vi "SCLN_GetResponseFromOldServer.vi"(2 "error in (no error)":errorcluster, 3 "Index for Server":i32) -> (0 "error out":errorcluster, 1 "Message":string)   [LabVIEW 2015]
uses:
  SCL_Header and Message.ctl
  SCL_Pending Action.ctl
  SCLN_RW_Select.ctl
panel:
  out "Pending Action":T1
  in  "Hdr-Msg":T2
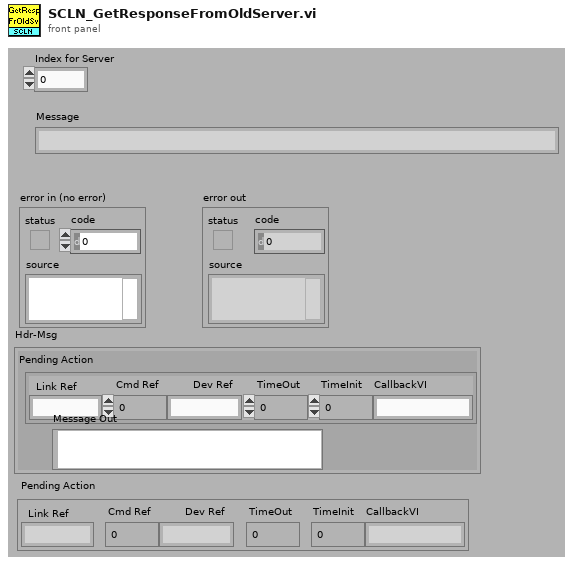
[diagram p1: front panel]
types:
  T1 = typedef "SCL_Pending Action.ctl" = cluster{"Cmd Ref":i32, "Dev Ref":string, "TimeOut":i32, "TimeInit":i32, "CallbackVI":string, "Link Ref":string}
  T2 = typedef "SCL_Header and Message.ctl" = cluster{"Pending Action":T1, "Message Out":string}
  T3 = typedef "SCLN_RW_Select.ctl" = enum16{"Read", "Write"}
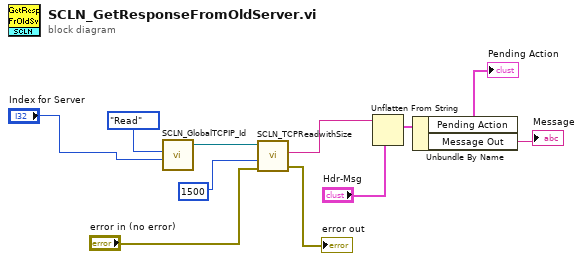
[diagram p0: block diagram]
diagram:
  n1 = call "SCLN_GlobalTCPIP_Id.vi"("Element"="Index for Server", "Operation"=SCLN_RW_Select."Read" ("GBL_RW")) -> ("TCPIP_Id Read"=w9:refnum<k5>)  [unwired: 2 in, 1 out]
  n2 = call "SCLN_TCPReadwithSize.vi"("error in (no error)"="error in (no error)", "timeout ms (600)"=1500, "connection ID"=w9) -> ("error out"=→"error out":errorcluster, "data out"=w5:string)  [unwired: 6 in, 1 out]
  n3 = Unflatten From String(type="Hdr-Msg", binary string=w5) -> (value=w3:T2)  [unwired: 3 in, 2 out]
  n4 = Unbundle By Name(w3) -> ("Pending Action"=→"Pending Action":T1, "Message Out"=→"Message":string)
